vi "prepDO_tt.vi"() -> ()   [LabVIEW 2015]
uses:
  <vilib>/DAQmx/write.llb/DAQmx Write (Digital 1D Wfm NChan NSamp).vi
  <vilib>/Waveform/DWDTOps.llb/DWDT Analog to Digital.vi
  <vilib>/DAQmx/create/channels.llb/DAQmx Create Channel (DO-Digital Output).vi
  <vilib>/DAQmx/configure/timing.llb/DAQmx Timing (Sample Clock).vi
  <vilib>/Waveform/DWDTOps.llb/DWDT Uncompress Digital.vi
  <vilib>/DAQmx/miscellaneous.llb/DAQmx Fill In Error Info.vi
panel:
  in  "error in":errorcluster
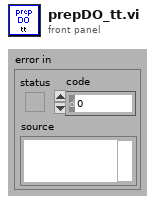
[diagram p1: front panel]
types:
  T1 = typedef "LVRectTypeDef.ctl" = cluster{"Left":i16, "Top":i16, "Right":i16, "Bottom":i16}
  T2 = cluster{"Xpixels":i32, "Vxminref":dbl, "Vxmaxref":dbl, "P":dbl, "Ypixels":i32, "Vyminref":dbl, "Vymaxref":dbl, "srate":sgl, "sAOxy":i32, "timeout":dbl, "type":string, "date":string, "time":string, "Colormap":u16, "Drawing Mode":u16, "Scanning Mode":u16, "square pixels":bool, "square matrix":bool, "Xpixels Img":i32, "Vx-min Img":dbl, "VX-max Img":dbl, "Ypixels Img":i32, "Vy-min Img":dbl, "Vy-max Img ":dbl, "Angle Img":dbl, "autoshutter":bool, "finite":bool, "cont":bool, "wavdet":bool, "measpoints":i32, "avpp":i32, "bufferAO":i32, "bufferAI":i32, "starttick":u32, "waveform":path, "Vx-ref":dbl, "Vy-ref":dbl, "refreshrate":dbl, "refreshbuffer":i32, "tt_cycles":i32, "motorref":refnum<k7>, "mirrorswitch":refnum<k7>, "sample mode":i32, "maxbufferAI":i32, "srateAODO":sgl, "bin":sgl, "Pel":sgl, "Angle draw":dbl, "srate Img":sgl, "ROIimg_plotbounds":T1, "auto OD":bool, "ODfilt":u16, "aAI":i32[], "aCI":i32[], "aAO":u32[], "aDO":u32[], "refwfsize":dbl, "Lifetime":bool, "Vz-Img":dbl, "Vz-ref":dbl, "Vz-reset":dbl, "AIoverride":bool}
  T3 = cluster{"StageS":i32, "StageL":i32, "currmeas data dir":path, "image OD":u16, "contour OD":u16, "point OD":u16, "AOlines":tag[], "AIlines":tag[], "CI lines":tag[], "DO lines":tag[], "AO names":string[], "CI names":string[], "AI names":string[], "DO names":string[], "CIextensions":string[], "AIextensions":string[], "Voltage to Ygalvo":i32, "Voltage to Xgalvo":i32, "Voltage to patch":i32, "640 shutter":i32, "2P shutter":i32, "LT timestamp":u32, "Vp":i32, "Ip":i32, "camera trigger":i32, "master data dir":path, "voltage to Zpos":i32, "Vto2P":i32, "640 AO":i32, "488 AO":i32, "532 AO":i32, "640TTL":u32, "488TTL":u32, "532TTL":u32, "Device 1 sampleclock out":tag, "Device 1 Starttrigger out":tag, "Device 2 sampleclock in":tag, "Device 2 StartTrigger in ":tag, "2PODTTL":u32, "488 shutter":u32, "LCVR red":u32, "LCVR blue":u32}
  T4 = cluster{"VtoP":sgl[], "CWlasers":sgl[], "shutter":sgl[], "488":sgl[], "532":sgl[], "640":sgl[], "LT marker":sgl[]}
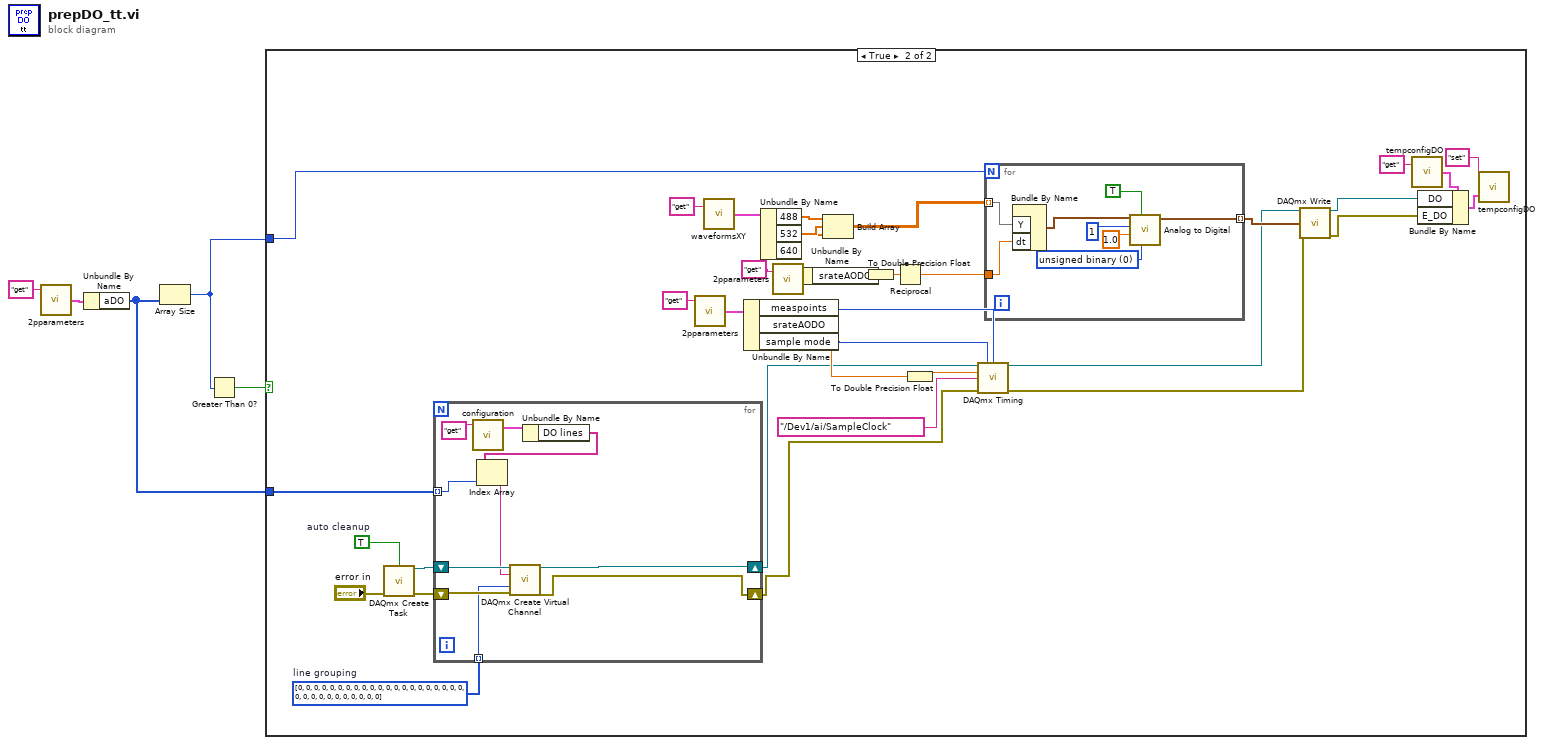
[diagram p0: block diagram]
diagram:
  n1 = call "2pparameters.vi"("command"="get") -> ("params out"=w4:T2)  [unwired: 1 in]
  n2 = Unbundle By Name(w4) -> ("aDO"=w3:u32[])
  n3 = Array Size(array=w3) -> (size(s)=w1:i32)
  n4 = Greater Than 0?(x=w1) -> (x > 0?=w2:bool)
  n5 = case shown="True" w2 {
    tunnel: w3 -> [_ w22]
    tunnel: w1 -> [_ w21]
    frame False {
    }
    frame True {
      w41 = i32[] [0, 0, 0, 0, 0, 0, 0, 0, 0, 0, 0, 0, 0, 0, 0, 0, 0, 0, 0, 0, 0, 0, 0, 0, 0, 0, 0, 0, 0, 0, 0, 0] items=["one channel for each line", "one channel for all lines"]  # line grouping
      w39 = TRUE  # auto cleanup
      n6 = call <vilib>:"DAQmx Create Task.vi"("auto cleanup"=w39, "error in"="error in") -> ("task out"=w40:refnum<k21>, "error out"=w38:errorcluster)  [unwired: 12 in]
      n7 = for {
        tunnel: w41 -> [w57] mode=indexing
        shift-right: [w50] -> w30
        shift-left: w38 -> [w58]
        tunnel: w22 -> [w54] mode=indexing
        shift-right: [w51] -> w31
        shift-left: w40 -> [w59]
        n8 = call "configuration.vi"("command"="get") -> ("config out"=w56:T3)  [unwired: 2 in, 1 out]
        n9 = Unbundle By Name(w56) -> ("DO lines"=w53:tag[])
        n10 = Index Array(array=w53, index=w54) -> (element=w52:tag)
        n11 = call-poly <vilib>:"DAQmx Create Virtual Channel.vi"("task in"=w59, "lines"=w52, "line grouping"=w57, "error in"=w58) -> ("task out"=w51:refnum<k21>, "error out"=w50:errorcluster)  [unwired: 10 in]
      }
      n12 = call "2pparameters.vi"("command"="get") -> ("params out"=w36:T2)  [unwired: 1 in]
      n13 = call "waveformsXY.vi"("command"="get") -> ("waveforms out"=w26:T4)  [unwired: 1 in]
      n14 = Unbundle By Name(w36) -> ("measpoints"=w29:i32, "srateAODO"=w32:sgl, "sample mode"=w28:i32)
      n15 = Unbundle By Name(w26) -> ("488"=w25:sgl[], "532"=w24:sgl[], "640"=w23:sgl[])
      n16 = call "2pparameters.vi"("command"="get") -> ("params out"=w17:T2)  [unwired: 1 in]
      n17 = Unbundle By Name(w17) -> ("srateAODO"=w19:sgl)
      n18 = Build Array(w25, w24, w23) -> (w20:sgl[][])
      n19 = To Double Precision Float(number=w19) -> (double precision float=w16:dbl)
      n20 = Reciprocal(x=w16) -> (1/x=w15:dbl)
      n21 = To Double Precision Float(number=w32) -> (double precision float=w34:dbl)
      n22 = call-poly <vilib>:"DAQmx Timing.vi"("task/channels in"=w31, "sample mode"=w28, "samples per channel"=w29, "rate"=w34, "source"=tag "/Dev1/ai/SampleClock", "error in"=w30) -> ("task out"=w13:refnum<k21>, "error out"=w12:errorcluster)  [unwired: 1 in, 7 out]
      n23 = for {
        N: w21 -> [_]
        tunnel: w20 -> [w49] mode=indexing
        tunnel: w15 -> [w48]
        tunnel: [w43] -> w14 mode=indexing
        w45 = u16 0 items=["unsigned binary", "offset binary", "2's complement"] ("data format (offset binary)")
        n24 = Bundle By Name("Y"=w49, "dt"=w48) -> (w44:waveform(sgl))  [unwired: 1 in]
        n25 = call-poly <vilib>:"Analog to Digital.vi"("data format (offset binary)"=w45, "compress digital (T)"=TRUE, "full-scale range (pk-pk)"=1.0, "resolution (16 bit)"=1, "analog waveform"=w44) -> ("digital waveform"=w43:digitalwaveform)  [unwired: 3 in, 3 out]
      }
      n26 = call-poly <vilib>:"DAQmx Write.vi"("task/channels in"=w13, "data"=w14, "error in"=w12) -> ("task out"=w8:refnum<k21>, "error out"=w7:errorcluster)  [unwired: 10 in, 1 out]
      n27 = call "tempconfigDO.vi"("command"="get") -> ("Temp Config out"=w10:cluster{"DO":refnum<k21>, "E_DO":errorcluster})  [unwired: 1 in]
      n28 = Bundle By Name(cluster=w10, "DO"=w8, "E_DO"=w7) -> (w6:cluster{"DO":refnum<k21>, "E_DO":errorcluster})
      n29 = call "tempconfigDO.vi"("Temp Config in"=w6, "command"="set") -> ()  [unwired: 1 out]
    }
  }
